vi "New.vi"(4 "Unescaped":bool, 6 "Delimiters":T1={"Close"="}}", "Open"="{{"}, 8 "Error In":errorcluster, 11 "Key":string) -> (0 "Error Out":errorcluster, 3 "Variable":refnum<class "Variable.lvclass">)   [LabVIEW 2018, in "Toolkit.lvlib" / "Nodes.lvlib" / "Variable.lvclass"]
doc: "Creates a new Variable node that represents a Mustache Escaped or Unescaped Variable tag in a parsed template."
uses:
  Variable.lvclass
  Type Definitions/Delimiters.ctl
  Variable.lvclass/Variable.ctl
  Toolkit.lvlib
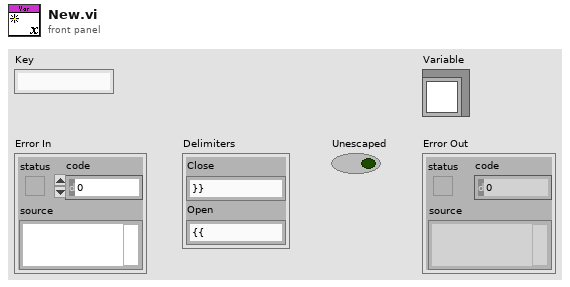
[diagram p1: front panel]
types:
  T1 = typedef "Toolkit.lvlib/Delimiters.ctl" = cluster{"Close":string, "Open":string}
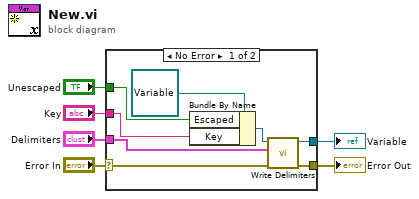
[diagram p0: block diagram]
diagram:
  n1 = case shown="No Error" "Error In" {
    selector: "Error In" -> [w8 w15]
    tunnel: "Key" -> [w14 _]
    tunnel: "Unescaped" -> [w13 _]
    tunnel: [w10 _] -> w4
    tunnel: [w9 w15] -> w3
    tunnel: "Delimiters" -> [w7 _]
    frame No Error {
      n2 = Bundle By Name(cluster=refnum<class "Variable.lvclass"> refnum ("Toolkit.lvlib:Nodes.lvlib:EscapedTag.lvclass"), "Escaped"=w13, "Key"=w14) -> (w12:refnum<class "Variable.lvclass">)
      n3 = call-dynamic "Write Delimiters.vi"("Error In"=w8, "Delimiters"=w7, "Node In"=w12) -> ("Error Out"=w9:errorcluster, "Node Out"=w10:refnum<class "Variable.lvclass">)  [unwired: 7 in]
    }
    frame Error {
    }
  }
  "Variable" <- w4
  "Error Out" <- w3
